vi "Base.vi"   [LabVIEW 2020, in "jettl.lvlib" / "Base jettl Actor.lvlib"]
uses:
  Base jettl Actor.lvlib
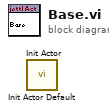
[diagram p0: block diagram]
diagram:
  n1 = call "Init Actor Default.vi"() -> ()  [unwired: 11 in, 1 out]
  n2 = call "Init Actor.vi"() -> ()  [unwired: 11 in, 1 out]
